vi "Enable Digital Bus Trigger Output.vi"(8 "error in (no error)":errorcluster, 10 "Enable Trigger Generate (F: Disable)":bool, 11 "VISA resource name":refnum<visa-resource-name>) -> (0 "error out":errorcluster, 3 "VISA resource name out":refnum<visa-resource-name>)   [LabVIEW 2020, in "Keysight E36300 Series.lvlib"]
doc: "Enables or disables bus-generated trigger signals on the digital pins.\n\n<b>Notes: </b>\n(1)This VI is only applicable for E36312A and E36313A models.\n(2)Pins 1 to 3 must be configured as trigger outputs before they can generate a trigger signal."
uses:
  Keysight E36300 Series.lvlib
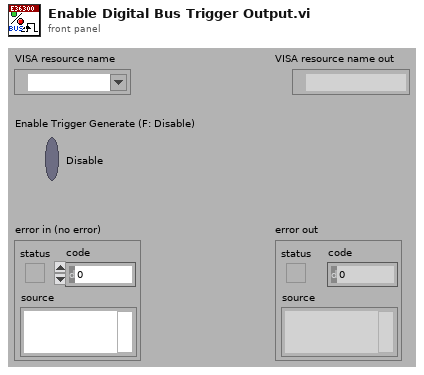
[diagram p1: front panel]
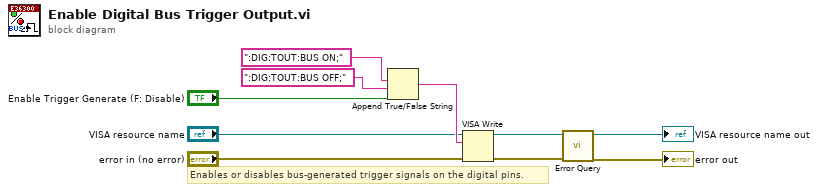
[diagram p0: block diagram]
diagram:
  # "Enables or disables bus-generated trigger signals on the digital pins."
  n1 = Append True/False String(1:"Enable Trigger Generate (F: Disable)", 2:":DIG:TOUT:BUS OFF;", 3:":DIG:TOUT:BUS ON;") -> (0:w7:string)  [unwired: 1 in]
  n2 = VISA Write(VISA resource name="VISA resource name", write buffer=w7, error in (no error)="error in (no error)") -> (VISA resource name out=w4:refnum<visa-resource-name>, error out=w3:errorcluster)  [unwired: 1 out]
  n3 = call "Error Query.vi"("error in (no error)"=w3, "VISA resource name"=w4) -> ("error out"=→"error out":errorcluster, "VISA resource name out"=→"VISA resource name out":refnum<visa-resource-name>)  [unwired: 6 in, 2 out]
